vi "Write CIFChannelMng.vi"(8 "error in (no error)":errorcluster, 10 "CIFChannelMng.lvclass":refnum<class "CIFChannelMng.lvclass">, 11 "CIFCorePlugin in":refnum<class "CIFCorePlugin.lvclass">) -> (0 "error out":errorcluster, 3 "CIFCorePlugin out":refnum<class "CIFCorePlugin.lvclass">)   [LabVIEW 2021, in "CIFCorePlugin.lvclass"]
uses:
  CIFCorePlugin.lvclass
  Channels/CIFChannelMng/CIFChannelMng.lvclass
  CIFCorePlugin.lvclass/CIFCorePlugin.ctl
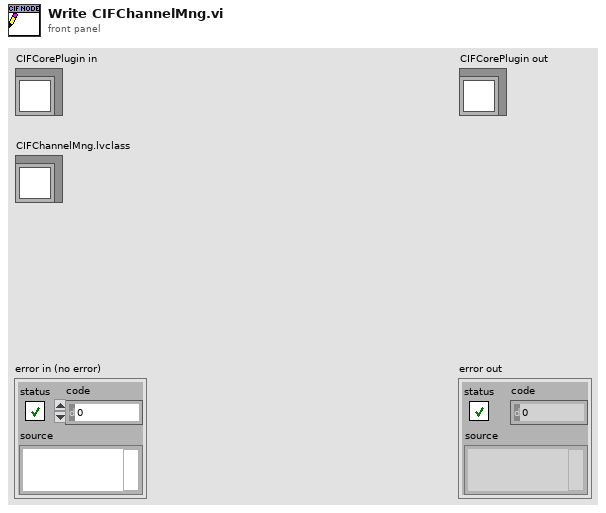
[diagram p1: front panel]
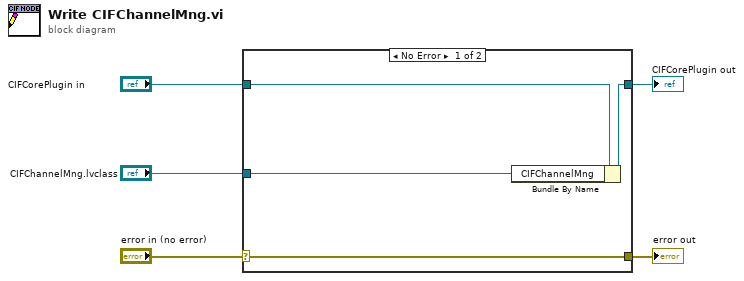
[diagram p0: block diagram]
diagram:
  n1 = case shown="No Error" "error in (no error)" {
    selector: "error in (no error)" -> [w9 w10]
    tunnel: [w9 w10] -> w4
    tunnel: [w7 w11] -> w2
    tunnel: "CIFCorePlugin in" -> [w8 w11]
    tunnel: "CIFChannelMng.lvclass" -> [w6 _]
    frame No Error {
      n2 = Bundle By Name(cluster=w8, "CIFChannelMng"=w6) -> (w7:refnum<class "CIFCorePlugin.lvclass">)
    }
    frame Error {
    }
  }
  "error out" <- w4
  "CIFCorePlugin out" <- w2
